vi "Do.vi"(8 "error in (no error)":errorcluster, 10 "Actor in":refnum<class "Actor.lvclass">, 11 "Close VISA Msg":refnum<class "Close VISA Msg.lvclass">) -> (0 "error out":errorcluster, 2 "Actor out":refnum<class "Actor.lvclass">)   [LabVIEW 2020, in "UI Actor.lvlib" / "Close VISA Msg.lvclass"]
doc: "This VI delivers the message to the actor by calling the appropriate method(s) on the actor."
uses:
  Close VISA Msg.lvclass
  <vilib>/ActorFramework/Actor/Actor.lvclass
  UI Actor/UI Actor.lvclass
  C:/Program Files/National Instruments/LabVIEW 2020/vi.lib/ActorFramework/Actor/Actor.lvclass
  03676969-acbb-4445-8d8f-d746683c63b4.vi
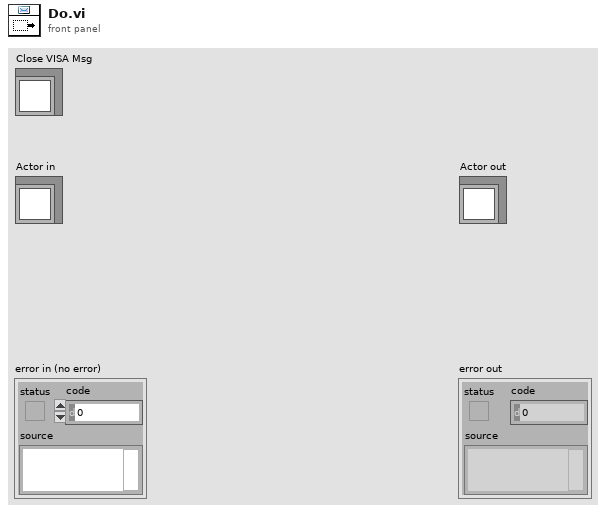
[diagram p1: front panel]
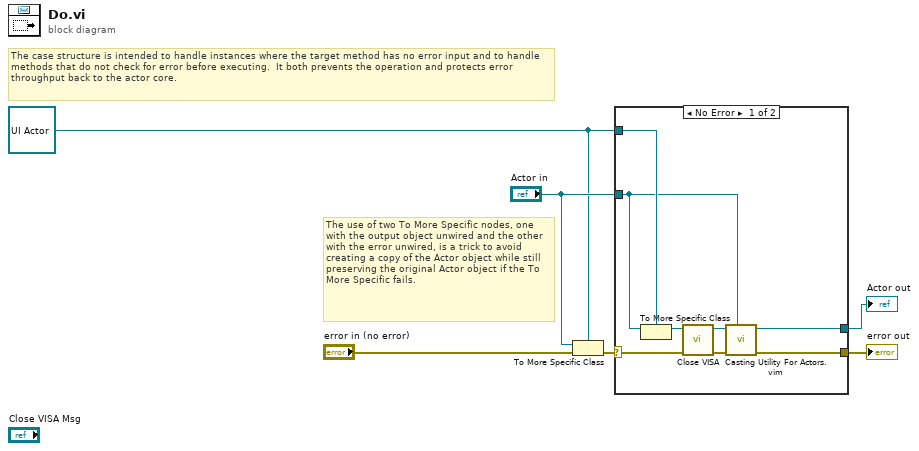
[diagram p0: block diagram]
diagram:
  w2 = refnum<class "UI Actor.lvclass"> refnum ("Actor in")
  # "The use of two To More Specific nodes, one with the output object unwired and the other with the error unwired, is a trick to avoid creating a copy of the Actor object while still preserving the original Actor object if the To More Specific fails."
  # "The case structure is intended to handle instances where the target method has no error input and to handle methods that do not check for error before executing.  It both prevents the operation and protects error throughput back to the actor core."
  n1 = To More Specific Class(target class=w2, reference="Actor in", error in="error in (no error)") -> (error out=w1:errorcluster)  [unwired: 1 out]
  n2 = case shown="No Error" w1 {
    selector: w1 -> [w14 w16]
    tunnel: [w8 w16] -> w6
    tunnel: [w9 w15] -> w5
    tunnel: "Actor in" -> [w11 w15]
    tunnel: w2 -> [w12 _]
    frame No Error {
      n3 = To More Specific Class(target class=w12, reference=w11) -> (specific class reference=w13:refnum<class "UI Actor.lvclass">)  [unwired: 1 in, 1 out]
      n4 = call "Close VISA.vi"("error in (no error)"=w14, "UI Actor in"=w13) -> ("error out"=w7:errorcluster, "UI Actor out"=w10:refnum<class "UI Actor.lvclass">)  [unwired: 8 in]
      n5 = call "Casting Utility For Actors.vim"("type"=w11, "error in (no error)"=w7, "Actor in"=w10) -> ("error out"=w8:errorcluster, "Actor out"=w9:refnum<class "Actor.lvclass">)  [unwired: 7 in]
    }
    frame Error {
      # "If type check fails, pass the original object out again."
    }
  }
  "error out" <- w6
  "Actor out" <- w5
